vi "ScanExperimentPaths.vi"(11 "Scan path":path) -> (3 "AvailableExperiments":T1[](array[typedef]))   [LabVIEW 2017]
uses:
  Types/ExperimentGrp.ctl
panel:
  in  "Cluster":T1
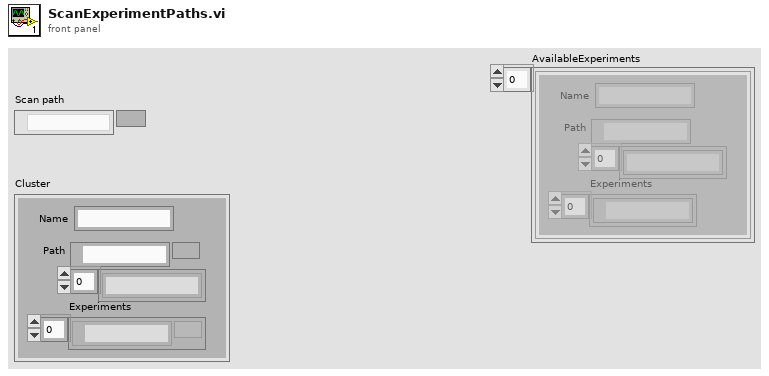
[diagram p1: front panel]
types:
  T1 = typedef "ExperimentGrp.ctl" = cluster{"Path":path, "Experiments":path[], "Name":string, "Experiment Names":string[]}
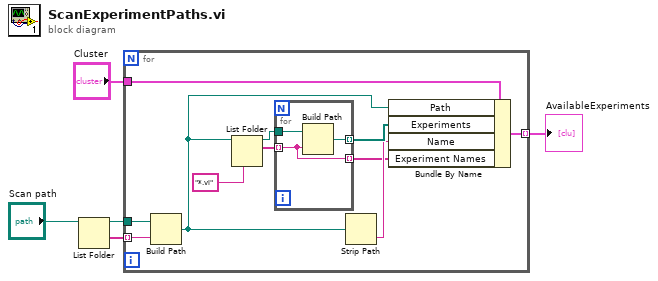
[diagram p0: block diagram]
diagram:
  n1 = List Folder(path="Scan path") -> (path out=w3:path, folder names=w4:string[])  [unwired: 3 in, 2 out]
  n2 = for {
    tunnel: w4 -> [w16] mode=indexing
    tunnel: w3 -> [w15]
    tunnel: [w10] -> w1 mode=indexing
    tunnel: "Cluster" -> [w9]
    n3 = Build Path(base path=w15, name or relative path=w16) -> (appended path=w8:path)
    n4 = List Folder(path=w8, pattern="*.vi") -> (path out=w14:path, filenames=w13:string[])  [unwired: 2 in, 2 out]
    n5 = for {
      tunnel: w14 -> [w18]
      tunnel: w13 -> [w17] mode=indexing
      tunnel: [w19] -> w11 mode=indexing
      tunnel: [w17] -> w6 mode=indexing
      n6 = Build Path(base path=w18, name or relative path=w17) -> (appended path=w19:path)
    }
    n7 = Strip Path(path=w8) -> (name=w7:string)  [unwired: 1 out]
    n8 = Bundle By Name(cluster=w9, "Path"=w8, "Experiments"=w11, "Name"=w7, "Experiment Names"=w6) -> (w10:T1)
  }
  "AvailableExperiments" <- w1
